vi "ciclofor_1.vi"() -> ()   [LabVIEW 2011]
panel:
  out "Potencia":dbl
  out "Exponente":dbl
  out "Base":dbl
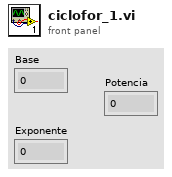
[diagram p1: front panel]
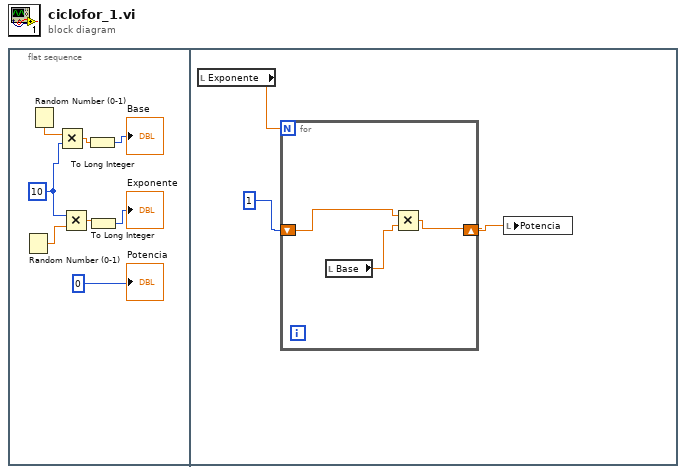
[diagram p0: block diagram]
diagram:
  n1 = flat-sequence {
    frame #0 {
      w6 = 10
      n2 = Random Number (0-1)() -> (number: 0 to 1=w7:dbl)
      n3 = Random Number (0-1)() -> (number: 0 to 1=w8:dbl)
      n4 = Multiply(x=w8, y=w6) -> (x*y=w5:dbl)
      n5 = Multiply(x=w6, y=w7) -> (x*y=w4:dbl)
      n6 = To Long Integer(number=w5) -> (32bit integer=→"Base":i32)
      n7 = To Long Integer(number=w4) -> (32bit integer=→"Exponente":i32)
      "Potencia" <- 0
    }
    frame #1 {
      n8 = local read "Exponente"() -> (w9:dbl)
      n9 = for {
        N: w9 -> [_]
        shift-right: [w12] -> w10
        shift-left: 1 -> [w14]
        n10 = local read "Base"() -> (w13:dbl)
        n11 = Multiply(x=w14, y=w13) -> (x*y=w12:dbl)
      }
      n12 = local write "Potencia"(w10) -> ()
    }
  }
